vi "chi.vi"(1 "g":u32, 2 "f":u32, 3 "e":u32) -> (0 "ch":u32)   [LabVIEW 2012, in "SHA256.lvlib"]
doc: "Computes the ch intermediate vairable in the compression phase of the SHA-256 algorithm"
uses:
  SHA256.lvlib
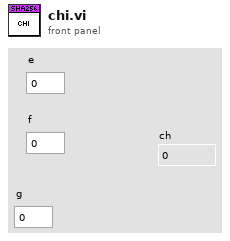
[diagram p1: front panel]
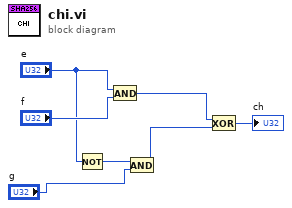
[diagram p0: block diagram]
diagram:
  n1 = Not(x="e") -> (.not. x?=w5:u32)
  n2 = And(x="e", y="f") -> (x .and. y?=w3:u32)
  n3 = And(x=w5, y="g") -> (x .and. y?=w2:u32)
  n4 = Exclusive Or(1:w2, 2:w3) -> (0:→"ch":u32)
